vi "iRobot PWM Low-Side Driver.vi"(0 "UART port in":T1, 5 "Low Side Driver 0 (0-128 duty cycle)":u8, 7 "Low Side Driver 1 (0-128 duty cycle)":u8, 9 "Low Side Driver 2 (0-128 duty cycle)":u8, 11 "error in":errorcluster) -> (4 "UART port out":T1, 15 "error out":errorcluster)   [LabVIEW 2010]
doc: "Set the PWM duty cycle of the low-side drivers.\n\nThis VI writes to, but does not read from, the serial port."
uses:
  UART/UART Port Type.ctl
  Open Interface Controls/iRobot OpCode.ctl
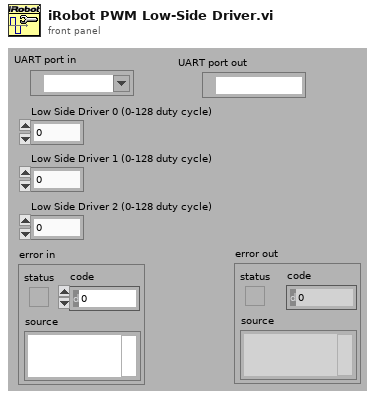
[diagram p1: front panel]
types:
  T1 = typedef "UART Port Type.ctl" = refnum<visa-resource-name>
  T2 = typedef "iRobot OpCode.ctl" = u8
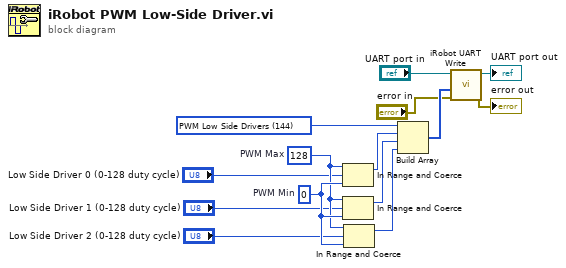
[diagram p0: block diagram]
diagram:
  w14 = u8 0  # PWM Min
  w9 = u8 128  # PWM Max
  w13 = T2 144 items=["Start"=128, "Baud"=129, "Control"=130, "Safe"=131, "Full"=132, "Demo"=136, "Demo - Cover"=135, "Demo - Cover and Dock"=143, "Demo - Spot"=134, "Drive"=137, "Drive Direct"=145, "LEDs"=139, "Digital Outputs"=147, "PWM Low Side Drivers"=144, "Low Side Drivers"=138, "Send IR"=151, "Song"=140, "Play Song"=141, "Sensors"=142, "Query List"=149, "Stream"=148, "Pause/Resume Stream"=150, "Script"=152, "Play Script"=153, "Show Script"=154, "Wait Time"=155, "Wait Distance"=156, "Wait Angle"=157, "Wait Event"=158] ("OpCode")
  n1 = In Range and Coerce(upper limit=w9, x="Low Side Driver 0 (0-128 duty cycle)", lower limit=w14) -> (coerced(x)=w12:u8)  [unwired: 1 out]
  n2 = In Range and Coerce(upper limit=w9, x="Low Side Driver 1 (0-128 duty cycle)", lower limit=w14) -> (coerced(x)=w11:u8)  [unwired: 1 out]
  n3 = In Range and Coerce(upper limit=w9, x="Low Side Driver 2 (0-128 duty cycle)", lower limit=w14) -> (coerced(x)=w10:u8)  [unwired: 1 out]
  n4 = Build Array(w13, w12, w11, w10) -> (w8:T2[])
  n5 = call "iRobot UART Write.vi"("error in"="error in", "data"=w8, "UART port in"="UART port in") -> ("error out"=→"error out":errorcluster, "UART port out"=→"UART port out":T1)  [unwired: 7 in]
